vi "Register Assert.vi"(4 "Unique ID":string, 6 "Call Chain":string[](array[string]), 7 "Execution time (s)":dbl=-1.0, 8 "error in (no error)":errorcluster, 9 "Succeeded":bool, 10 "Message":string, 11 "Test Manager in":refnum<class "Test Manager.lvclass">) -> (0 "error out":errorcluster, 3 "Test Manager out":refnum<class "Test Manager.lvclass">)   [LabVIEW 2013, in "Caraya.lvlib" / "Test Manager.lvclass"]
uses:
  Test Manager.lvclass
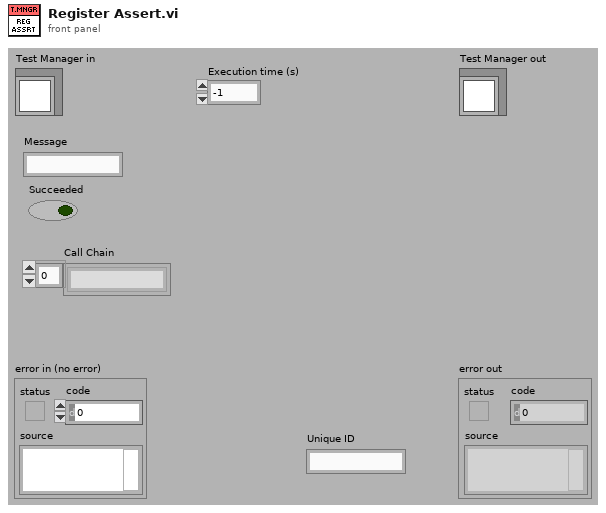
[diagram p1: front panel]
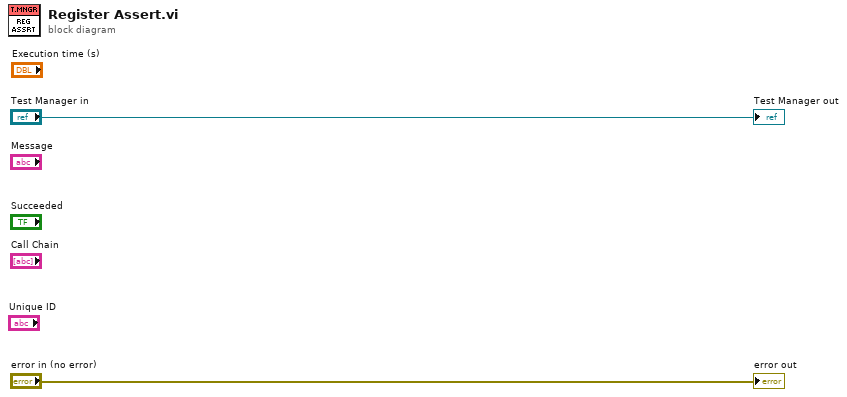
[diagram p0: block diagram]
diagram:
  "error out" <- "error in (no error)"
  "Test Manager out" <- "Test Manager in"
